vi "Train_GetDataForTraining.vi"(7 "DataIn":bool, 8 "error in (no error)":errorcluster, 9 "WR":dbl, 10 "Wl":dbl, 11 "robot body ref":refnum<k20>) -> (0 "error out":errorcluster, 3 "Data":dbl[][](array[numeric]))   [LabVIEW 2017]
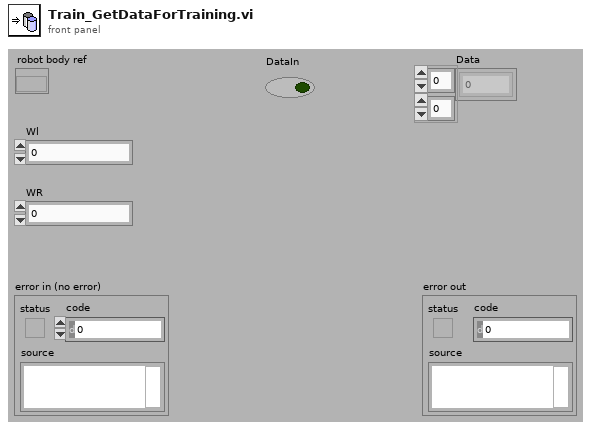
[diagram p1: front panel]
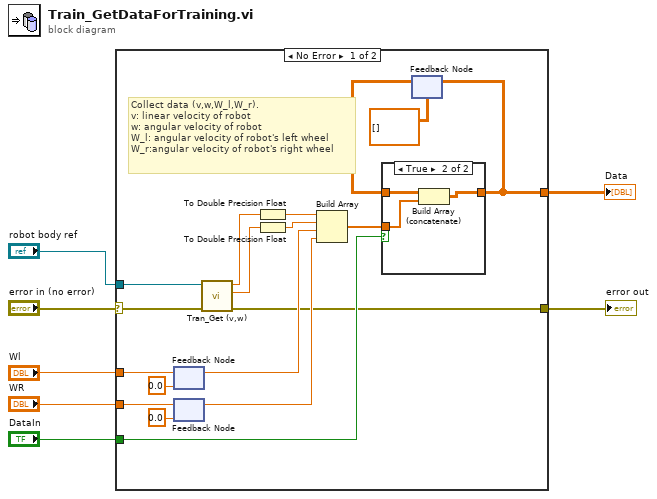
[diagram p0: block diagram]
diagram:
  n1 = case shown="No Error" "error in (no error)" {
    selector: "error in (no error)" -> [w12 w30]
    tunnel: "robot body ref" -> [w25 _]
    tunnel: "Wl" -> [w22 _]
    tunnel: "WR" -> [w21 _]
    tunnel: "DataIn" -> [w17 _]
    tunnel: [w16 _] -> w3
    tunnel: [w13 w30] -> w2
    frame No Error {
      # "Collect data (v,w,W_l,W_r).\nv: linear velocity of robot\nw: angular velocity of robot\nW_l: angular velocity of robot's left wheel\nW_r:angular velocity of robot's right wheel"
      n2 = feedback #1(0.0) -> (w20:dbl)
      n3 = feedback-in #1(w22) -> ()
      n4 = feedback #2(0.0) -> (w19:dbl)
      n5 = feedback-in #2(w21) -> ()
      n6 = call "Tran_Get (v,w).vi"("error in (no error)"=w12, "robot body ref"=w25) -> ("error out"=w13:errorcluster, "Angular Veloctiy"=w8:sgl, "Linear Velocity"=w11:sgl)  [unwired: 7 in]
      n7 = To Double Precision Float(number=w11) -> (double precision float=w10:dbl)
      n8 = To Double Precision Float(number=w8) -> (double precision float=w9:dbl)
      n9 = Build Array(w10, w9, w20, w19) -> (w18:dbl[])
      n10 = feedback #3(dbl[][] []) -> (w15:dbl[][])
      n11 = case shown="True" w17 {
        tunnel: w18 -> [_ w29]
        tunnel: [w26 w28] -> w16
        tunnel: w15 -> [w26 w27]
        frame False {
        }
        frame True {
          n12 = Build Array (concatenate)(w27, w29) -> (w28:dbl[][])
        }
      }
      n13 = feedback-in #3(w16) -> ()
    }
    frame Error {
    }
  }
  "Data" <- w3
  "error out" <- w2
